vi "VFH-read_folder-LabVIEW.vi"(10 "Folder Path":path) -> (0 "Samples":i32, 1 "size(s)":i32, 2 "avg output":T1)   [LabVIEW 2020, in "VFH-VNA_File_Handler.lvlib"]
uses:
  VFH-VNA_File_Handler.lvlib
  VFH-file_cluster-LabVIEWVNA.ctl
panel:
  out "Array 5":dbl[][](array[numeric])
  out "Array 4":dbl[](array[numeric])
  out "Array 3":dbl[][](array[numeric])
  out "Array":T1[](array[typedef])
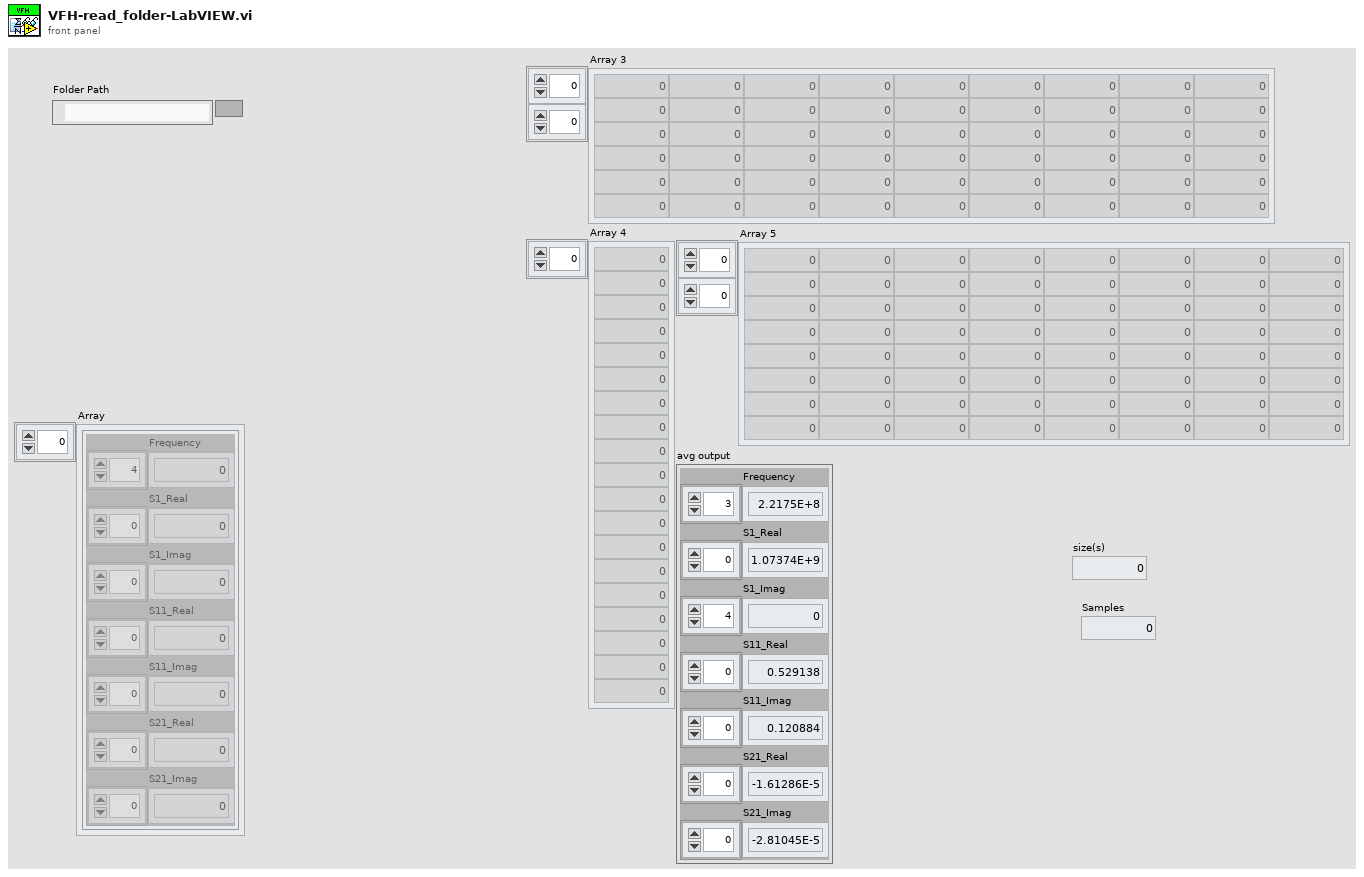
[diagram p1: front panel]
types:
  T1 = typedef "VFH-VNA_File_Handler.lvlib/VFH-file_cluster-LabVIEWVNA.ctl" = cluster{"Frequency":dbl[], "S1_Real":dbl[], "S1_Imag":dbl[], "S11_Real":dbl[], "S11_Imag":dbl[], "S21_Real":dbl[], "S21_Imag":dbl[]}
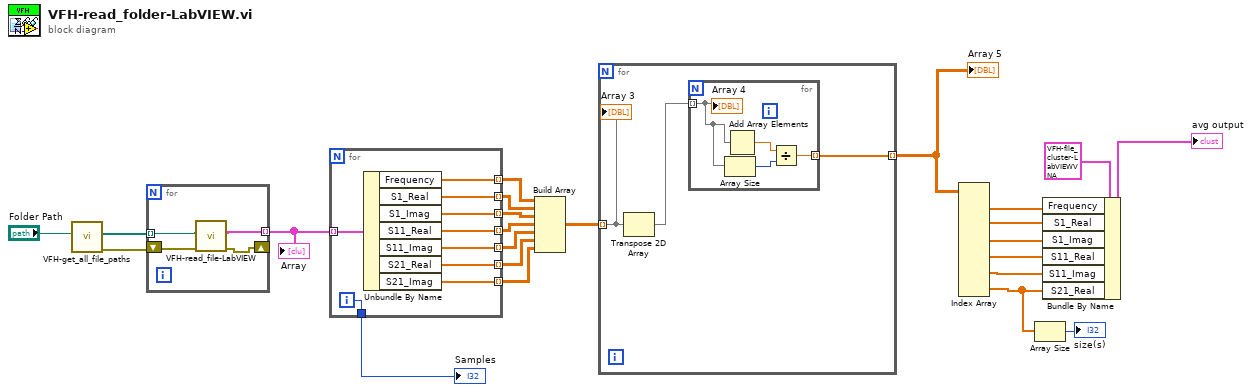
[diagram p0: block diagram]
diagram:
  n1 = call "VFH-get_all_file_paths.vi"("Folder Path"="Folder Path") -> ("error out"=w22:errorcluster, "All Files in Dir"=w21:path[])  [unwired: 8 in, 1 out]
  n2 = for {
    shift-right: [w24] -> _
    shift-left: w22 -> [w26]
    tunnel: w21 -> [w27] mode=indexing
    tunnel: [w25] -> w20 mode=indexing
    n3 = call "VFH-read_file-LabVIEW.vi"("error in"=w26, "file path (dialog if empty)"=w27) -> ("error out"=w24:errorcluster, "output cluster"=w25:T1)  [unwired: 8 in]
  }
  "Array" <- w20
  n4 = for {
    tunnel: w20 -> [w36] mode=indexing
    tunnel: [w35] -> w19 mode=indexing
    tunnel: [w34] -> w18 mode=indexing
    tunnel: [w33] -> w17 mode=indexing
    tunnel: [w32] -> w16 mode=indexing
    tunnel: [w31] -> w15 mode=indexing
    tunnel: [w30] -> w14 mode=indexing
    tunnel: [w29] -> w13 mode=indexing
    tunnel: [w28] -> w3
    i -> [w28]
    n5 = Unbundle By Name(w36) -> ("Frequency"=w35:dbl[], "S1_Real"=w34:dbl[], "S1_Imag"=w33:dbl[], "S11_Real"=w32:dbl[], "S11_Imag"=w31:dbl[], "S21_Real"=w30:dbl[], "S21_Imag"=w29:dbl[])
  }
  "Samples" <- w3
  n6 = Build Array(w19, w18, w17, w16, w15, w14, w13) -> (w12:dbl[][][])
  n7 = for {
    tunnel: w12 -> [w39] mode=indexing
    tunnel: [w37] -> w11 mode=indexing
    n8 = Transpose 2D Array(2D array=w39) -> (transposed array=w38:dbl[][])
    n9 = for {
      tunnel: w38 -> [w41] mode=indexing
      tunnel: [w40] -> w37 mode=indexing
      n10 = Array Size(array=w41) -> (size(s)=w43:i32)
      n11 = Add Array Elements(numeric array=w41) -> (sum=w42:dbl)
      n12 = Divide(x=w42, y=w43) -> (x/y=w40:dbl)
      "Array 4" <- w41
    }
    "Array 3" <- w39
  }
  "Array 5" <- w11
  n13 = Index Array(array=w11) -> (element #1=w8:dbl[], element #2=w7:dbl[], element #3=w6:dbl[], element #4=w5:dbl[], element #5=w4:dbl[], element #6=w2:dbl[])  [unwired: 12 in]
  n14 = Array Size(array=w2) -> (size(s)=→"size(s)":i32)
  n15 = Bundle By Name(cluster=T1 {"Frequency"=array[802 elements], "S1_Real"=array[802 elements], "S1_Imag"=array[802 elements], "S11_Real"=array[802 elements], "S11_Imag"=array[802 elements], "S21_Real"=array[802 elements], "S21_Imag"=array[802 elements]} ("output cluster"), "Frequency"=w8, "S1_Real"=w7, "S1_Imag"=w6, "S11_Real"=w5, "S11_Imag"=w4, "S21_Real"=w2) -> (→"avg output":T1)
